vi "Realtime Struct for ADS1015.vi"() -> ()   [LabVIEW 2014]
uses:
  <vilib>/Platform/TimedLoop/XDataNode/timing_clust.ctl
  <vilib>/Platform/TimedLoop/XDataNode/nitl_modes.ctl
  <vilib>/Platform/TimedLoop/XDataNode/wakeup.ctl
  <vilib>/platform/TimedLoop/XDataNode/XDataNode.xnode
  <vilib>/Platform/TimedLoop/XDataNode/XDNodeRunTimeDep.lvlib
panel:
  in  "Stop":bool
  in  "Amplitude":dbl(slide)=5.0 scale=0.0..10.0
  out "Result Data":dbl(graph)
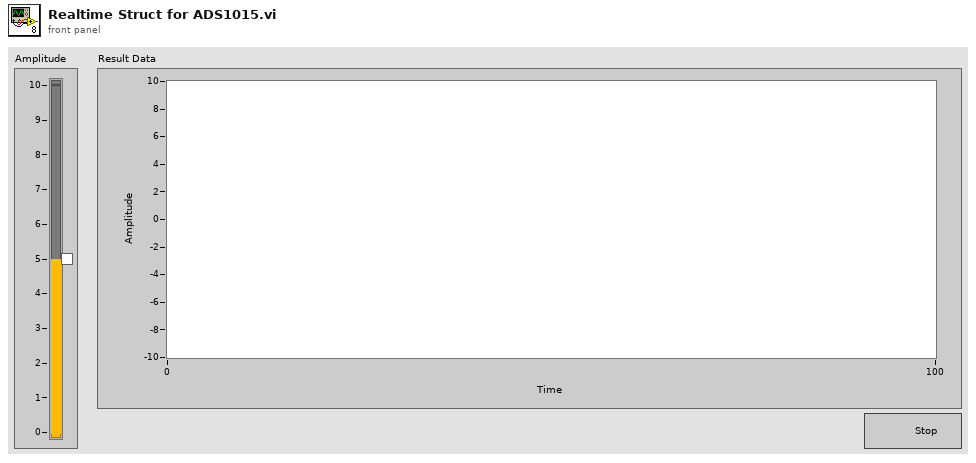
[diagram p1: front panel]
types:
  T1 = typedef "XDNodeRunTimeDep.lvlib/timing_clust.ctl" = cluster{"Expected End [f-1]":u64, "Actual End [f-1]":u64, "Finished Late? [f-1]":bool, "Expected End [i-1]":u64, "Actual End [i-1]":u64, "Finished Late? [i-1]":bool, "Expected Start [i]":u64, "Actual Start [i]":u64, "Expected Start [f]":u64, "Actual Start [f]":u64, "Source Name":string, "Structure Name":string, "Period":i64, "Deadline":i64, "Offset":i64, "Start":i64, "Priority":i32, "Timeout":i32, "Mode":T2, "Wakeup Reason":T3, "Error":errorcluster, "Source Type":string, "Secondary Source Type":string, "Global End Time":u64, "Global Start Time":u64, "Frame Duration":u64, "Iteration Duration":u64, "Assigned CPU":i32, "I/O Scan Engine Mode":u32}
  T2 = typedef "XDNodeRunTimeDep.lvlib/nitl_modes.ctl" = enum32{"No Change", "Process missed periods, maintain original phase", "Discard missed periods, maintain original phase", "Process missed periods, ignore original phase", "Discard missed periods, ignore original phase"}
  T3 = typedef "XDNodeRunTimeDep.lvlib/wakeup.ctl" = enum32{"Normal", "Aborted", "Asynchronous wakeup", "Timing source error", "Timed loop error", "Timeout"}
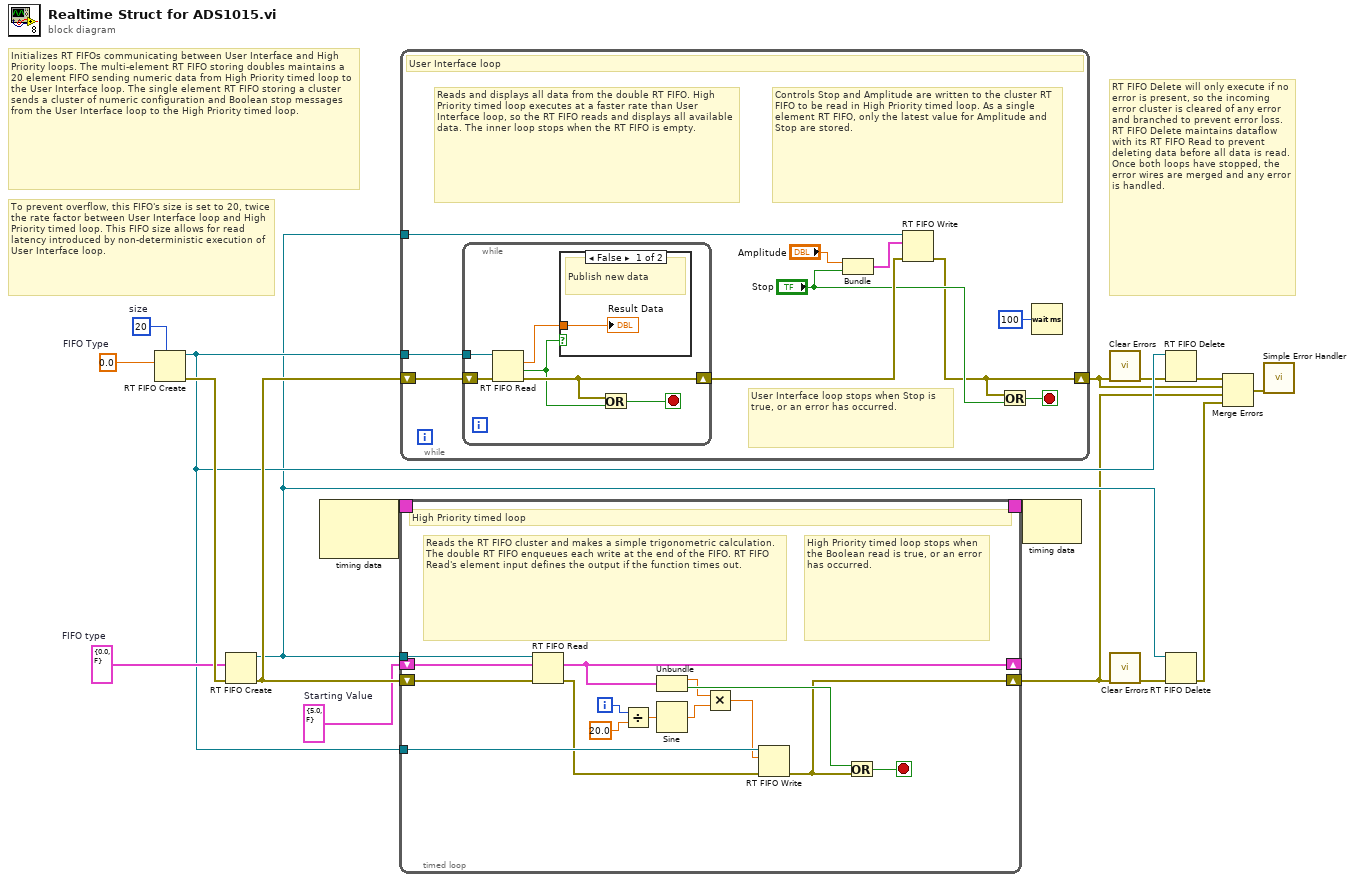
[diagram p0: block diagram]
diagram:
  w1 = 0.0  # FIFO Type
  w11 = cluster{dbl, bool} {5.0, FALSE}  # Starting Value
  w12 = cluster{dbl, bool} {0.0, FALSE}  # FIFO type
  w13 = u32 20  # size
  # "RT FIFO Delete will only execute if no error is present, so the incoming error cluster is cleared of any error and branched to prevent error loss. RT FIFO Delete maintains dataflow with its RT FIFO Read to prevent deleting data before all data is read. Once both loops have stopped, the error wires are merged and any error is handled."
  # "To prevent overflow, this FIFO's size is set to 20, twice the rate factor between User Interface loop and High Priority timed loop. This FIFO size allows for read latency introduced by non-deterministic execution of User Interface loop."
  # "Initializes RT FIFOs communicating between User Interface and High Priority loops. The multi-element RT FIFO storing doubles maintains a 20 element FIFO sending numeric data from High Priority timed loop to the User Interface loop. The single element RT FIFO storing a cluster sends a cluster of numeric configuration and Boolean stop messages from the User Interface loop to the High Priority timed loop."
  n1 = RT FIFO Create(1:w1, 4:w13) -> (8:w10:refnum<k33>, 11:w15:errorcluster)  [unwired: 3 in, 4 out]
  n2 = RT FIFO Create(1:w12, 3:w15) -> (8:w9:refnum<k33>, 11:w14:errorcluster)  [unwired: 3 in, 4 out]
  n3 = node-c288() -> (w17:T1)  [unwired: 1 in, 1 out]
  n4 = timed-loop "High Priority timed loop" {
    shift-left: w11 -> [w31]
    shift-right: [w26] -> _
    shift-right: [w18] -> w4
    shift-left: w14 -> [w28]
    timing: w17 -> [_]
    timing-out: [_] -> w16
    tunnel: w9 -> [w32]
    tunnel: w10 -> [w30]
    i -> [w27]
    stop <- w24 stop-if-true
    # "Reads the RT FIFO cluster and makes a simple trigonometric calculation. The double RT FIFO enqueues each write at the end of the FIFO. RT FIFO Read's element input defines the output if the function times out."
    # "High Priority timed loop stops when the Boolean read is true, or an error has occurred."
    # "High Priority timed loop"
    n5 = RT FIFO Read(0:w32, 1:w31, 3:w28) -> (9:w26:cluster{dbl, bool}, 11:w29:errorcluster)  [unwired: 4 out]
    n6 = Divide(x=w27, y=20.0) -> (x/y=w22:dbl)
    n7 = Unbundle(w26) -> (w20:dbl, w25:bool)
    n8 = Sine(x=w22) -> (sin(x)=w21:dbl)
    n9 = Multiply(x=w20, y=w21) -> (x*y=w19:dbl)
    n10 = RT FIFO Write(0:w30, 1:w19, 3:w29) -> (11:w18:errorcluster)  [unwired: 1 in, 4 out]
    n11 = Or(x=w25, y=w18) -> (x .or. y?=w24:bool)
  }
  n12 = while "User Interface loop" {
    shift-right: [w35] -> w5
    shift-left: w14 -> [w43]
    tunnel: w9 -> [w42]
    tunnel: w10 -> [w44]
    stop <- w40 stop-if-true
    # "User Interface loop stops when Stop is true, or an error has occurred."
    # "Controls Stop and Amplitude are written to the cluster RT FIFO to be read in High Priority timed loop. As a single element RT FIFO, only the latest value for Amplitude and Stop are stored."
    # "Reads and displays all data from the double RT FIFO. High Priority timed loop executes at a faster rate than User Interface loop, so the RT FIFO reads and displays all available data. The inner loop stops when the RT FIFO is empty."
    # "User Interface loop"
    n13 = while {
      tunnel: w44 -> [w50]
      shift-right: [w46] -> w41
      shift-left: w43 -> [w49]
      stop <- w47 stop-if-true
      n14 = RT FIFO Read(0:w50, 3:w49) -> (9:w48:dbl, 10:w45:bool, 11:w46:errorcluster)  [unwired: 1 in, 3 out]
      n15 = case shown="False" w45 {
        tunnel: w48 -> [w51 _]
        frame False {
          # "Publish new data"
          "Result Data" <- w51
        }
        frame True {
          # "No new data"
        }
      }
      n16 = Or(x=w46, y=w45) -> (x .or. y?=w47:bool)
    }
    n17 = Bundle("Amplitude"="Amplitude", "Stop"="Stop") -> (w37:cluster{"Amplitude":dbl, "Stop":bool})  [unwired: 1 in]
    n18 = RT FIFO Write(0:w42, 1:w37, 3:w41) -> (11:w35:errorcluster)  [unwired: 2 in, 3 out]
    n19 = Or(x=w35, y="Stop") -> (x .or. y?=w40:bool)
    n20 = Wait (ms)(milliseconds to wait=u32 100 ("millisecond multiple")) -> ()  [unwired: 1 out]
  }
  n21 = node-c288(w16) -> ()  [unwired: 1 out]
  n22 = call <vilib>:"Clear Errors.vi"("error in (no error)"=w5) -> ("error out"=w7:errorcluster)  [unwired: 5 in, 1 out]
  n23 = call <vilib>:"Clear Errors.vi"("error in (no error)"=w4) -> ("error out"=w8:errorcluster)  [unwired: 5 in, 1 out]
  n24 = RT FIFO Delete(0:w10, 3:w7) -> (11:w6:errorcluster)  [unwired: 1 in]
  n25 = RT FIFO Delete(0:w9, 3:w8) -> (11:w3:errorcluster)  [unwired: 1 in]
  n26 = Merge Errors(w6, w5, w4, w3) -> (w2:errorcluster)
  n27 = call <vilib>:"Simple Error Handler.vi"("error in (no error)"=w2) -> ()  [unwired: 4 in, 5 out]
